vi "Disk Usage.vi"(8 "error in (no error)":errorcluster, 11 "System Status Actor in":refnum<class "System Status Actor.lvclass">) -> (0 "error out":errorcluster, 3 "System Status Actor out":refnum<class "System Status Actor.lvclass">)   [LabVIEW 2020, in "RTAF.lvlib" / "System Status Actor.lvclass"]
uses:
  System Status Actor.lvclass
panel:
  out "Total [MB]":dbl
  out "Used [MB]":dbl
  out "df | grep /dev/root":string
  out "Free [MB]":dbl
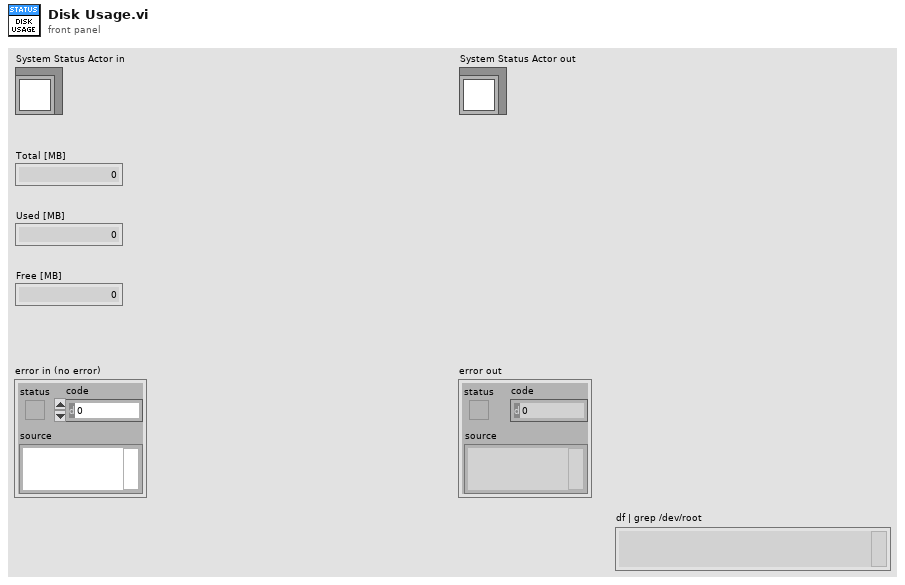
[diagram p1: front panel]
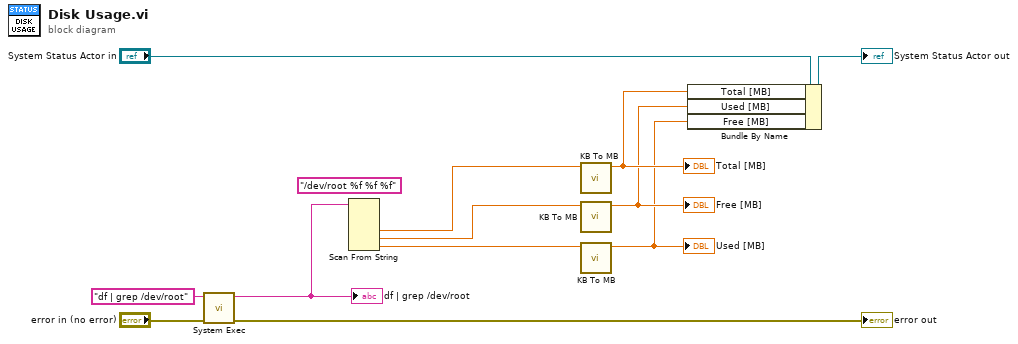
[diagram p0: block diagram]
diagram:
  (unwired) "/dev/root %f %f %f" ("format string")
  n1 = call <vilib>:"System Exec.vi"("error in (no error)"="error in (no error)", "command line"="df | grep /dev/root") -> ("error out"=→"error out":errorcluster, "standard output"=w4:string)  [unwired: 6 in, 2 out]
  "df | grep /dev/root" <- w4
  n2 = Scan From String(input string=w4) -> (output 1=w3:dbl, output 2=w2:dbl, output 3=w1:dbl)  [unwired: 6 in, 3 out]
  n3 = call "KB To MB.vi"("KB"=w3) -> ("MB"=w9:dbl)  [unwired: 10 in]
  "Total [MB]" <- w9
  n4 = call "KB To MB.vi"("KB"=w2) -> ("MB"=w8:dbl)  [unwired: 10 in]
  "Free [MB]" <- w8
  n5 = call "KB To MB.vi"("KB"=w1) -> ("MB"=w7:dbl)  [unwired: 10 in]
  "Used [MB]" <- w7
  n6 = Bundle By Name(cluster="System Status Actor in", "Total [MB]"=w9, "Used [MB]"=w8, "Free [MB]"=w7) -> (→"System Status Actor out":refnum<class "System Status Actor.lvclass">)
